vi "sub_get_token_for_device.vi"(8 "error in (no error)":errorcluster, 11 "daq.io type in":T1={"daq.io ref"=refnum, "daq.io API Base"="http://dashboard.daq.io/api/v1", "Device Key"="", "Account ID"="", "online"=TRUE, "SSL"=FALSE}) -> (0 "error out":errorcluster, 1 "Device ID":string, 2 "Token ID":string, 3 "daq.io type out":T1={"daq.io ref"=refnum, "daq.io API Base"="http://dashboard.daq.io/api/v1", "Device Key"="", "Account ID"="", "online"=TRUE, "SSL"=FALSE})   [LabVIEW 2013, in "daqio minimal.lvlib"]
doc: "This VI returns the currently associated Token ID and the Device ID for a specified Device"
uses:
  daqio minimal.lvlib
  _typedefs/daqio-Type.ctl
  <vilib>/httpClient/ClientHandle.ctl
  <vilib>/Easy HTTP Client/Easy HTTP.lvlib
  <vilib>/httpClient/LabVIEWHTTPClient.lvlib
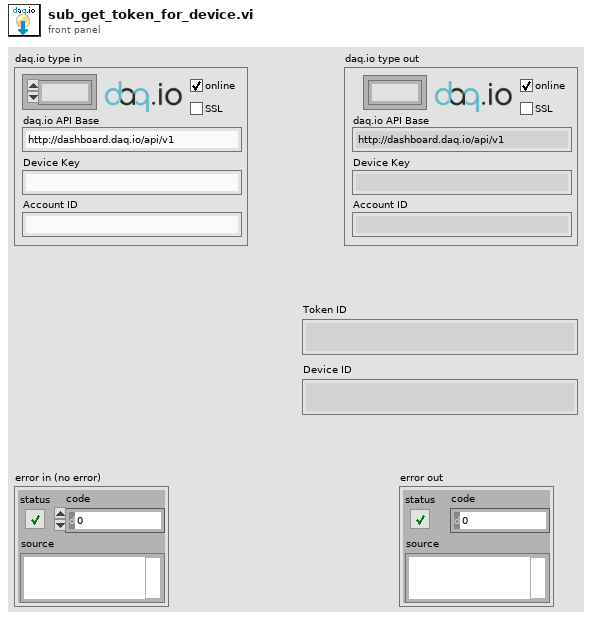
[diagram p1: front panel]
types:
  T1 = typedef "daqio minimal.lvlib/daqio-Type.ctl" = cluster{"daq.io ref":T2, "daq.io API Base":string, "Device Key":string, "Account ID":string, "online":bool, "SSL":bool}
  T2 = typedef "LabVIEWHTTPClient.lvlib/ClientHandle.ctl" = refnum<k1>
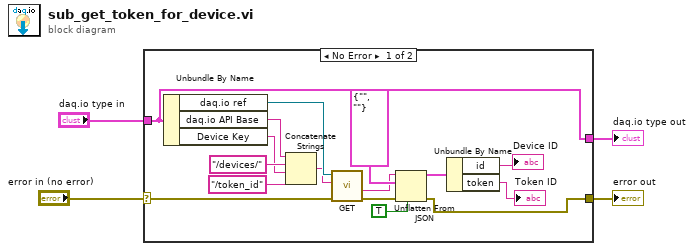
[diagram p0: block diagram]
diagram:
  n1 = case shown="No Error" "error in (no error)" {
    selector: "error in (no error)" -> [w15 w21]
    tunnel: [w5 w21] -> w3
    tunnel: "daq.io type in" -> [w14 w22]
    tunnel: [w14 w22] -> w1
    frame No Error {
      n2 = Unbundle By Name(w14) -> ("daq.io ref"=w20:T2, "daq.io API Base"=w19:string, "Device Key"=w17:string)
      n3 = Concatenate Strings(w19, "/devices/" ("string"), w17, "/token_id" ("string")) -> (w16:string)
      n4 = call <vilib>:"GET.vi"("error in (no error)"=w15, "url"=w16, "client handle"=w20) -> ("error out"=w10:errorcluster, "body"=w11:string)  [unwired: 4 in, 3 out]
      n5 = Unflatten From JSON(JSON string=w11, type and defaults=cluster{"id":string, "token":string} {"id"="", "token"=""}, default null elements? (F)=TRUE, error in (no error)=w10) -> (value=w8:cluster{"id":string, "token":string}, error out=w5:errorcluster)  [unwired: 3 in]
      n6 = Unbundle By Name(w8) -> ("id"=→"Device ID":string, "token"=→"Token ID":string)
    }
    frame Error {
    }
  }
  "error out" <- w3
  "daq.io type out" <- w1
